vi "Enable Range Lock.vi"(7 "Range Lock Enabled (F: Disabled)":bool, 8 "error in (no error)":errorcluster, 11 "VISA resource name":refnum<visa-resource-name>) -> (0 "error out":errorcluster, 3 "VISA resource name out":refnum<visa-resource-name>)   [LabVIEW 2012, in "Fluke 5080.lvlib"]
doc: "Sets whether or not locks in the present range, or selects auto ranging for DC Voltage and DC Current single outputs."
uses:
  <instrlib>/Fluke 5080/Fluke 5080.lvlib
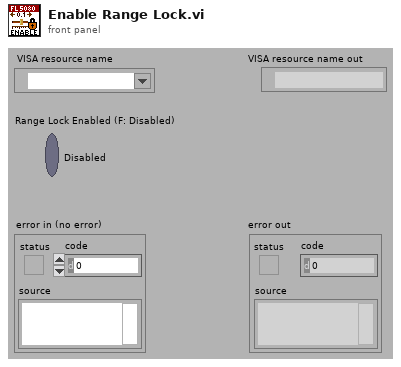
[diagram p1: front panel]
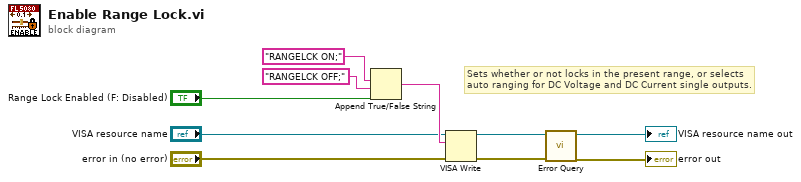
[diagram p0: block diagram]
diagram:
  # "Sets whether or not locks in the present range, or selects\nauto ranging for DC Voltage and DC Current single outputs."
  n1 = Append True/False String(1:"Range Lock Enabled (F: Disabled)", 2:"RANGELCK OFF;", 3:"RANGELCK ON;") -> (0:w7:string)  [unwired: 1 out]
  n2 = VISA Write(VISA resource name="VISA resource name", write buffer=w7, error in (no error)="error in (no error)") -> (VISA resource name out=w4:refnum<visa-resource-name>, error out=w3:errorcluster)  [unwired: 1 out]
  n3 = call <instrlib>:"Error Query.vi"("error in (no error)"=w3, "VISA resource name"=w4) -> ("error out"=→"error out":errorcluster, "VISA resource name out"=→"VISA resource name out":refnum<visa-resource-name>)  [unwired: 8 out]
